vi "Filter Empties.vi"(10 "In":string[](array[string])) -> (2 "Out":string[](array[string]))   [LabVIEW 2013]
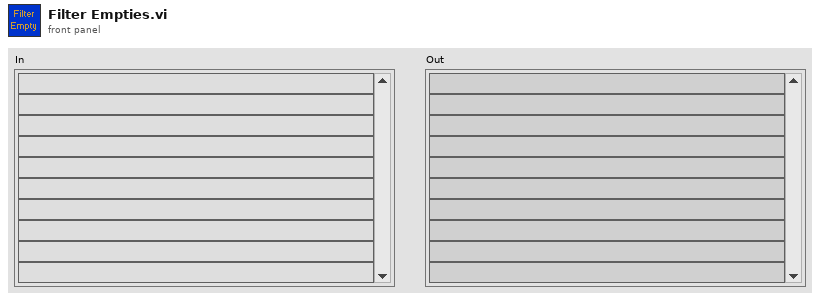
[diagram p1: front panel]
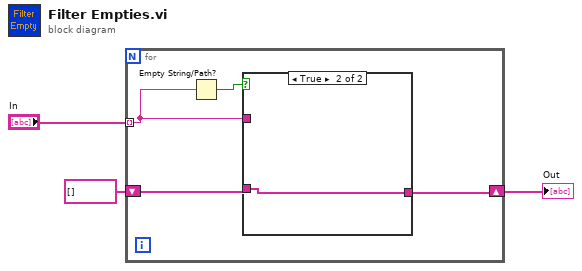
[diagram p0: block diagram]
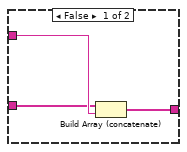
[diagram p2: hidden frame]
diagram:
  n1 = for {
    tunnel: "In" -> [w6] mode=indexing
    shift-right: [w5] -> w1
    shift-left: string[] [] -> [w4]
    n2 = Empty String/Path?(string/path=w6) -> (empty?=w7:bool)
    n3 = case shown="True" w7 {
      tunnel: w6 -> [w10 _]
      tunnel: [w9 w11] -> w5
      tunnel: w4 -> [w8 w11]
      frame False {
        n4 = Build Array (concatenate)(w8, w10) -> (w9:string[])
      }
      frame True {
      }
    }
  }
  "Out" <- w1
